vi "hatchPanelLoop.vi"() -> ()   [LabVIEW 2018]
uses:
  <vilib>/Platform/TimedLoop/XDataNode/timing_clust.ctl
  <vilib>/Platform/TimedLoop/XDataNode/nitl_modes.ctl
  <vilib>/Platform/TimedLoop/XDataNode/wakeup.ctl
  hatchPanelEnum.ctl
  HatchPanelMotionEnum.ctl
  HatchGrabPistonEnum.ctl
  hatchPanelNotifierCluster.ctl
  hatchPanelLockEnum.ctl
  hatchPanelStatemachineEnum.ctl
  stachModeHatchPanelStatemachineEnum.ctl
  hatchPanelClimbSMEnum.ctl
  <vilib>/platform/TimedLoop/XDataNode/XDataNode.xnode
  <vilib>/Platform/TimedLoop/XDataNode/XDNodeRunTimeDep.lvlib
  <userlib>/836-Library/System/TDMS_V2/Support/TDMS_DevRef.ctl
  <userlib>/836-Library/System/TDMS_V2/Support/Logging_Settings.ctl
  <userlib>/836-Library/System/TDMS_V2/Support/Group_FIFO_Config.ctl
  <userlib>/836-Library/System/TDMS_V2/Support/Channel_FIFO_Config.ctl
panel:
  in  "Tab Control":enum32{"Stach/OG", "Climb"}(tab)
  in  "hatchPanelSMGatherExtendTime":u32=380
  in  "hatchPanelSMScoreExtendTime":u32=700
  in  "hatchPanelSMGatherRetractTime":u32=650
  in  "hatchPanelSMScoreRetract":u32=500
  in  "hatchPanelSMReleaseTime":u32=150
  in  "hatchPanelSMGrabTime":u32=80
  in  "hatchPanelSMUnlockTime":u32=20
  in  "DistanceWantedFromTarget(Inch)":dbl=8.0
  in  "DistanceWantedAwayFromLoadingStation":dbl=-24.0
  out "Encoder Inches":dbl=-27.864021650326798
  in  "PanelDistanceDetect(V)":dbl=1.1
  in  "Wait for Unlock Time (ms)":u32=200
  in  "Wait for Extend Time (ms)":u32=1000
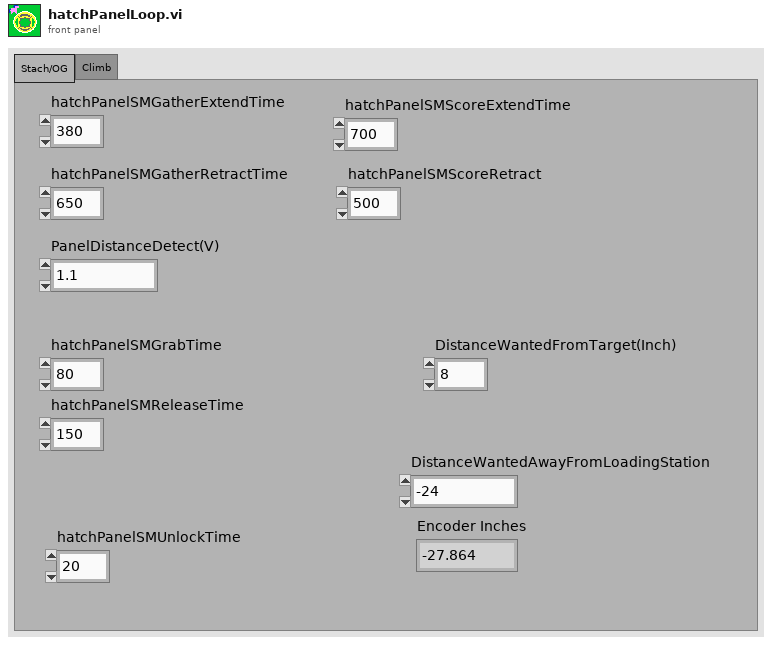
[diagram p1: front panel]
types:
  T1 = typedef "XDNodeRunTimeDep.lvlib/timing_clust.ctl" = cluster{"Expected End [f-1]":u64, "Actual End [f-1]":u64, "Finished Late? [f-1]":bool, "Expected End [i-1]":u64, "Actual End [i-1]":u64, "Finished Late? [i-1]":bool, "Expected Start [i]":u64, "Actual Start [i]":u64, "Expected Start [f]":u64, "Actual Start [f]":u64, "Source Name":string, "Structure Name":string, "Period":i64, "Deadline":i64, "Offset":i64, "Start":i64, "Priority":i32, "Timeout":i32, "Mode":T2, "Wakeup Reason":T3, "Error":errorcluster, "Source Type":string, "Secondary Source Type":string, "Global End Time":u64, "Global Start Time":u64, "Frame Duration":u64, "Iteration Duration":u64, "Assigned CPU":i32, "I/O Scan Engine Mode":u32}
  T2 = typedef "XDNodeRunTimeDep.lvlib/nitl_modes.ctl" = enum32{"No Change", "Process missed periods, maintain original phase", "Discard missed periods, maintain original phase", "Process missed periods, ignore original phase", "Discard missed periods, ignore original phase"}
  T3 = typedef "XDNodeRunTimeDep.lvlib/wakeup.ctl" = enum32{"Normal", "Aborted", "Asynchronous wakeup", "Timing source error", "Timed loop error", "Timeout"}
  T4 = typedef "WPI_SolenoidDevRef.ctl" = cluster{"DevStatus":errorcluster, "Pneumatics Control Module":u8, "Forward Solenoid Channel":T5, "Reverse Solenoid Channel":T5}
  T5 = typedef "WPI_SolenoidChannel.ctl" = enum8{"Solenoid 0", "Solenoid 1", "Solenoid 2", "Solenoid 3", "Solenoid 4", "Solenoid 5", "Solenoid 6", "Solenoid 7", "Invalid"}
  T6 = typedef "HatchGrabPistonEnum.ctl" = enum16{"Open", "Close"}
  T7 = typedef "HatchPanelMotionEnum.ctl" = enum16{"Retract", "Extend"}
  T8 = typedef "hatchPanelEnum.ctl" = enum16{"do nothing", "State Machine", "Stach Mode", "Climb Mode", "Retracted Closed", "Retracted Open", "Extended Closed", "Extended Open"}
  T9 = typedef "hatchPanelLockEnum.ctl" = enum16{"Unlocked", "Locked "}
  T10 = typedef "hatchPanelStatemachineEnum.ctl" = enum16{"Open to Gather", "Wait for Gather Extend", "Gather Extended", "Wait for Grab Panel", "Grab Panel", "Closed to Score", "Wait for Score Extend", "Ready to Score ", "Wait for Release Panel", "Release Panel", "Wait for Gather Retract", "Wait for Score Retract", "Wait for Gather Unlock", "Wait for Score Unlock", "Wait for Score Retract (Lock)", "Wait for Gather Retract (Lock)", "Gather End Lock", "Score End Lock"}
  T11 = typedef "stachModeHatchPanelStatemachineEnum.ctl" = enum16{"Stach Open to Gather", "Stach Wait for Gather Extend", "Stach Gather Extended", "Stach Wait for Grab Panel", "Stach Grab Panel", "Stach Closed to Score", "Stach Wait for Sonar Signal", "Stach Wait for Score Extend", "Stach Ready to Score ", "Stach Wait for Release Panel", "Stach Release Panel", "Stach Wait for Gather Retract", "Stach Wait for Score Retract", "Stach Wait for Gather Unlock", "Stach Wait for Score Unlock"}
  T12 = enum16{"Stach Open to Gather", "Stach Wait for Gather Extend", "Stach Gather Extended", "Stach Wait for Grab Panel", "Stach Grab Panel", "Stach Closed to Score", "Stach Wait for Sonar Signal", "Stach Wait for Score Extend", "Stach Ready to Score ", "Stach Wait for Release Panel", "Stach Release Panel", "Stach Wait for Gather Retract", "Stach Wait for Score Retract", "Stach Wait for Gather Unlock", "Stach Wait for Score Unlock", "Stach Gather End Lock", "Stach Score End Lock"}
  T13 = typedef "hatchPanelClimbSMEnum.ctl" = enum16{"Start", "Unlock", "Extend", "Ready for Climb", "Finished Climb"}
  T14 = typedef "hatchPanelNotifierCluster.ctl" = cluster{"Hatch Panel State":T8, "Mechanism Motion":bool, "Gathering Claw Motion":bool, "Scoring Claw Motion":bool}
  T15 = typedef "TDMS_DevRef.ctl" = cluster{"Name":string, "File Ref":refnum<k34>, "Start Time":timestamp, "Logging Settings":T16, "Group FIFO Config":T17[], "Data To Write":refnum<data-value>, "semaphore":T19, "Ref Time Reset":refnum<k4>}
  T16 = typedef "Logging_Settings.ctl" = cluster{"Data Grab Period":dbl, "File Write Period":dbl, "Max Stored Size":dbl, "Burst Size":dbl}
  T17 = typedef "Group_FIFO_Config.ctl" = cluster{"Group":string, "Channels":T18[], "Channel Names":string[]}
  T18 = typedef "Channel_FIFO_Config.ctl" = cluster{"Channel":string, "FIFO":refnum<k33>}
  T19 = typedef "Semaphore RefNum" = refnum<k1>
  T20 = typedef "WPI_MotorControlDeviceRef.ctl" = cluster{"DeviceStatus":errorcluster, "Type":T21, "PWM":cluster{"PWM Channel":T22, "DeadBand":T23}, "CAN":cluster{"Device Number":u8, "SetOutput VI Ref":variant, "GetOutput VI Ref":variant, "Enable VI Ref":variant, "Disable VI Ref":variant, "Data":variant}, "Invert":bool, "DIO PWM":cluster{"PWM \"Enable\" Channel":T22, "DIOChannel":T24, "PWM Rate":dbl}}
  T21 = typedef "WPI_MotorControlType.ctl" = enum16{"PWM", "CAN", "DIO PWM"}
  T22 = typedef "FPGA_DIOPWMChannel.ctl" = enum8{"PWM 0", "PWM 1", "PWM 2", "PWM 3", "PWM 4", "PWM 5", "PWM 6", "PWM 7", "PWM 8", "PWM 9", "PWM MXP 0", "PWM MXP 1", "PWM MXP 2", "PWM MXP 3", "PWM MXP 4", "PWM MXP 5", "PWM MXP 6", "PWM MXP 7", "PWM MXP 8", "PWM MXP 9", "Invalid"}
  T23 = typedef "WPI_PWMDeadband.ctl" = cluster{"Name":string, "maxPositivePwm":i32, "minPositivePwm":i32, "centerPwm":i32, "maxNegativePwm":i32, "minNegativePwm":i32, "angularRange":u16}
  T24 = typedef "FPGA_DIOChannel.ctl" = enum8{"DIO 0", "DIO 1", "DIO 2", "DIO 3", "DIO 4", "DIO 5", "DIO 6", "DIO 7", "DIO 8", "DIO 9", "DIO MXP 0", "DIO MXP 1", "DIO MXP 2", "DIO MXP 3", "DIO MXP 4", "DIO MXP 5", "DIO MXP 6", "DIO MXP 7", "DIO MXP 8", "DIO MXP 9", "DIO MXP 10", "DIO MXP 11", "DIO MXP 12", "DIO MXP 13", "DIO MXP 14", "DIO MXP 15", "SPI Port CS1", "SPI Port CS2", "SPI Port CS3", "SPI Port MISO", "SPI Port MOSI", "Invalid"}
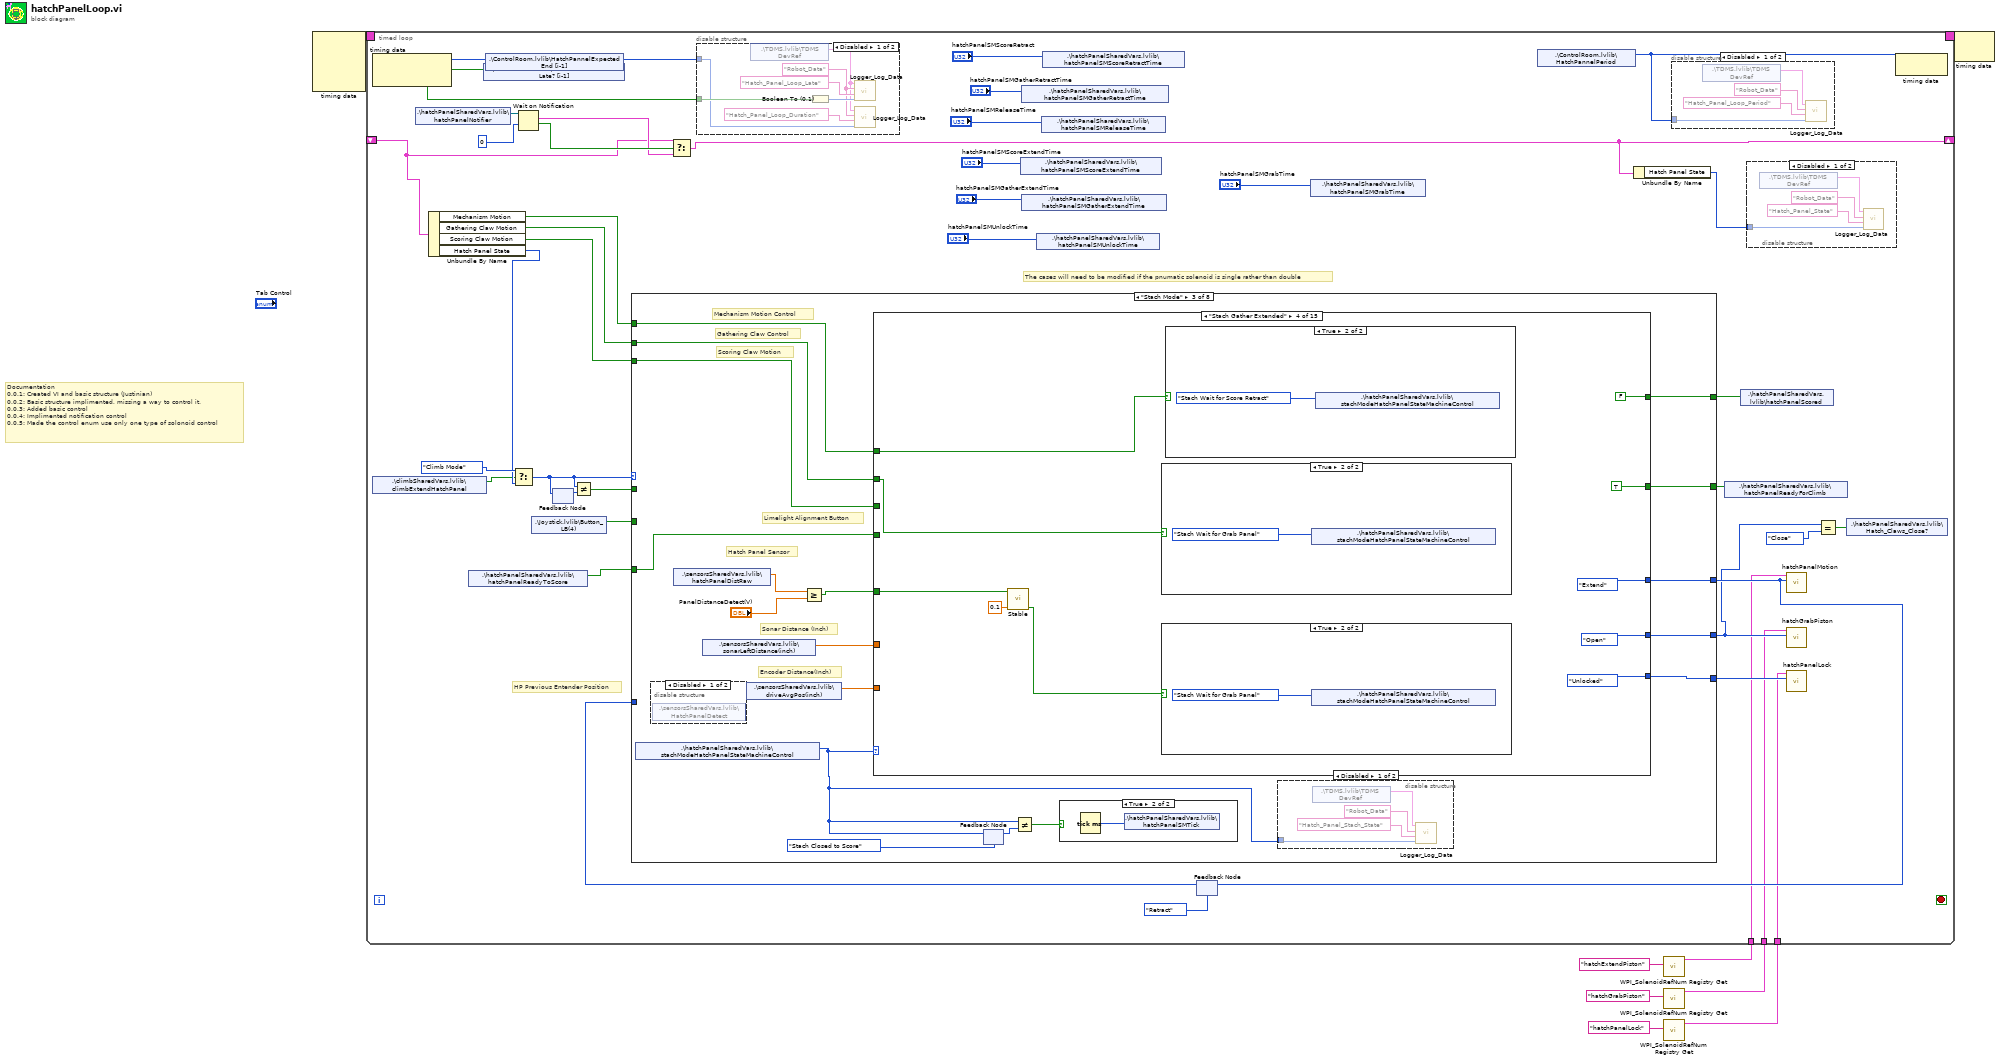
[diagram p0: block diagram]
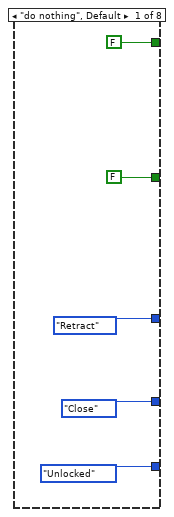
[diagram p5: hidden frame]
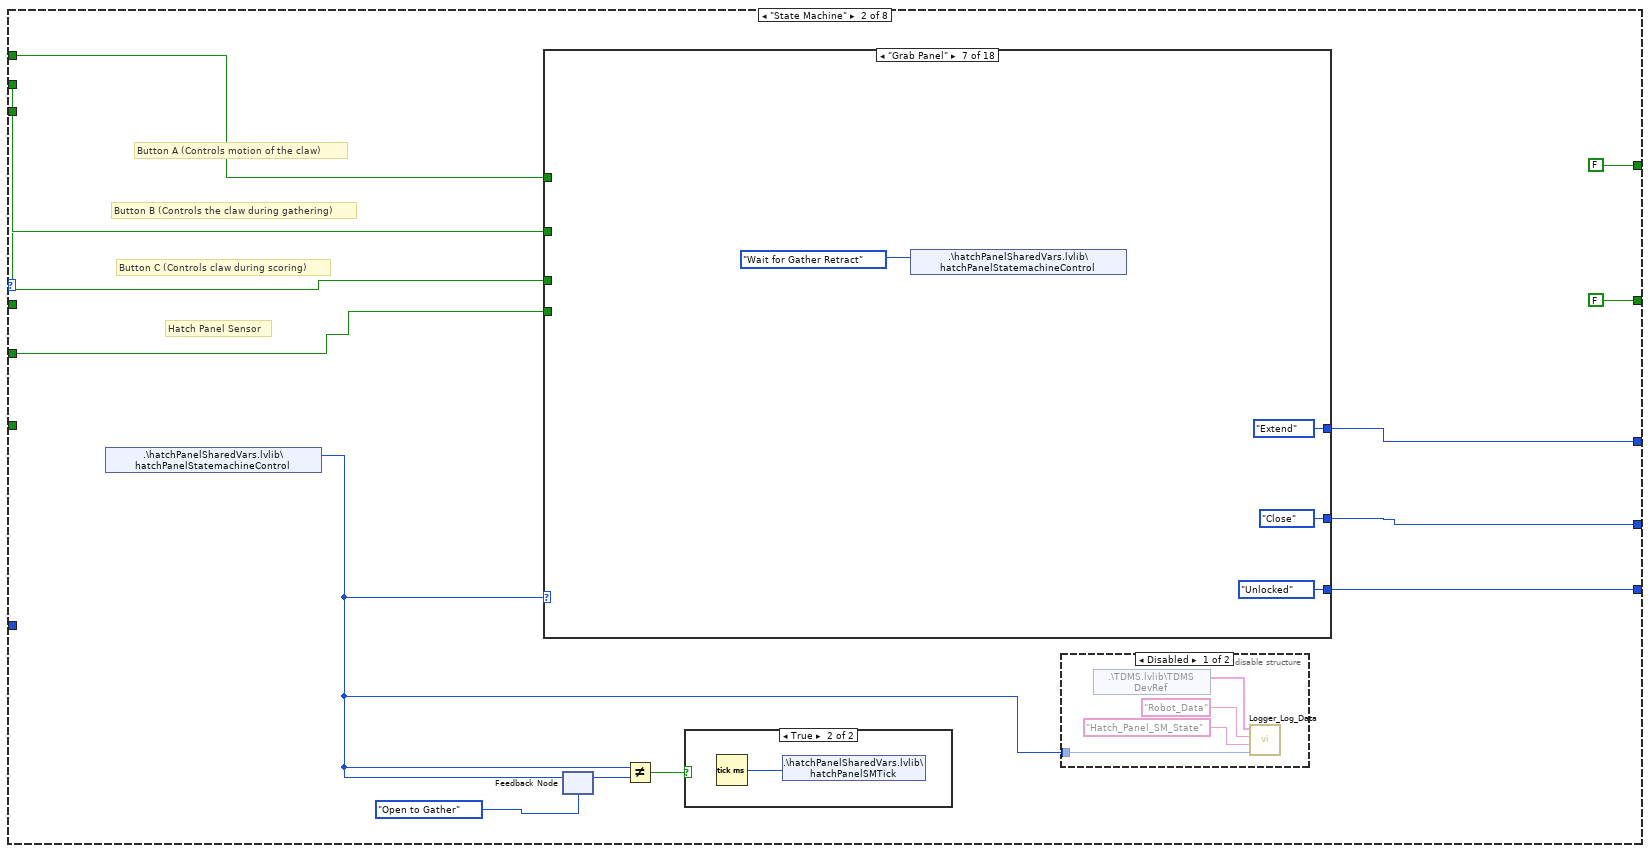
[diagram p6: hidden frame]
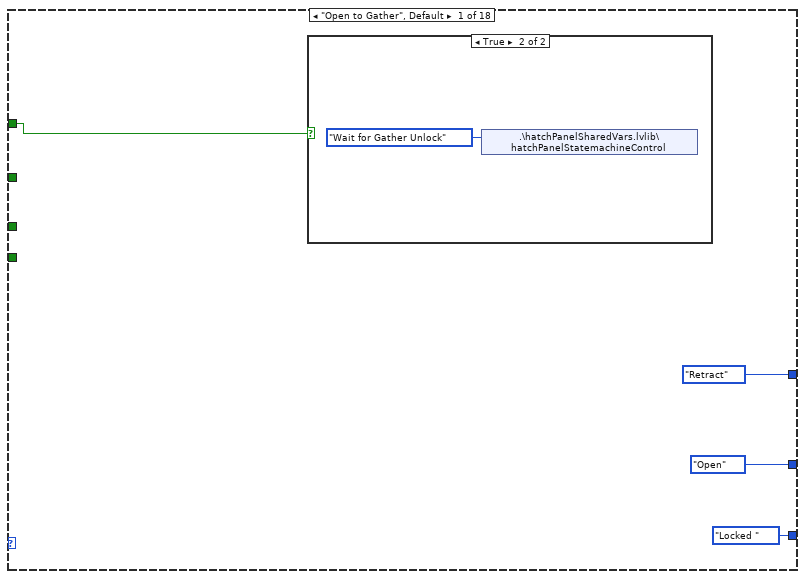
[diagram p9: hidden frame]
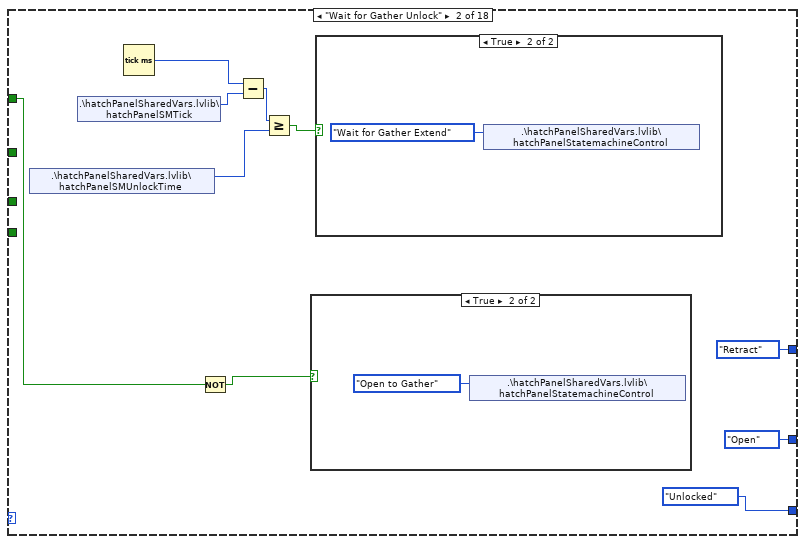
[diagram p11: hidden frame]
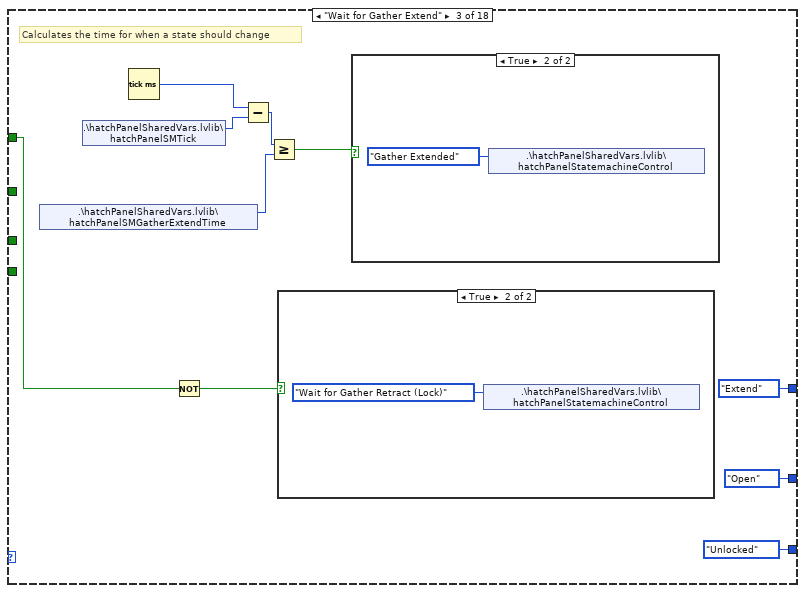
[diagram p14: hidden frame]
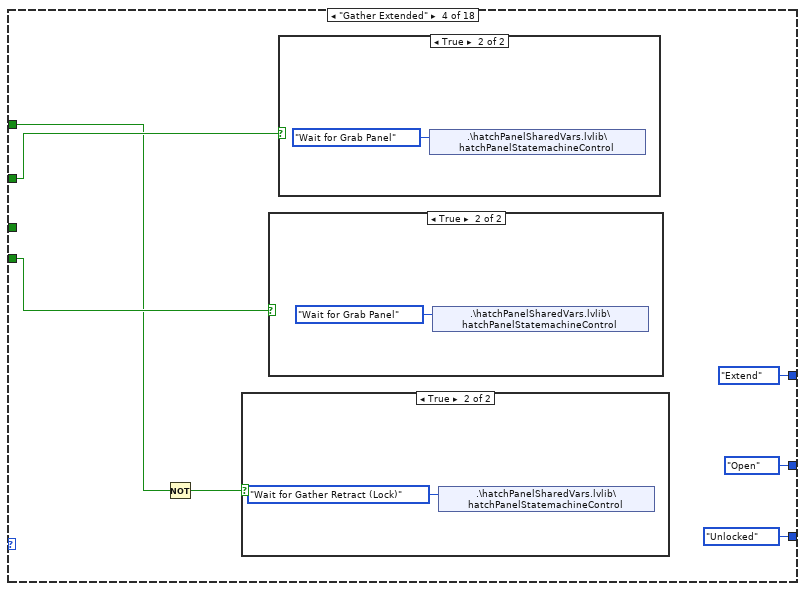
[diagram p17: hidden frame]
diagram:
  # "Documentation\n0.0.1: Created VI and basic structure (Justinian)\n0.0.2: Basic structure implimented, missing a way to control it.\n0.0.3: Added basic control\n0.0.4: Implimented notification control\n0.0.5: Made the control enum use only one type of solonoid control"
  n1 = node-c288() -> (w8:T1)  [unwired: 4 in]
  n2 = call <vilib>:"WPI_SolenoidRefNum Registry Get.vi"("refnum name"="hatchExtendPiston") -> ("SolenoidDevRef"=w3:T4)  [unwired: 9 in, 1 out]
  n3 = call <vilib>:"WPI_SolenoidRefNum Registry Get.vi"("refnum name"="hatchGrabPiston") -> ("SolenoidDevRef"=w2:T4)  [unwired: 9 in, 1 out]
  n4 = call <vilib>:"WPI_SolenoidRefNum Registry Get.vi"("refnum name"="hatchPanelLock") -> ("SolenoidDevRef"=w1:T4)  [unwired: 9 in, 1 out]
  n5 = timed-loop {
    timing: w8 -> [_]
    timing-out: [_] -> w7
    shift-right: [w17] -> _
    shift-left: _ -> [w18]
    tunnel: w3 -> [w12]
    tunnel: w2 -> [w11]
    tunnel: w1 -> [w10]
    stop <- _ stop-if-true
    # "HP Previous Entender Position"
    # "The cases will need to be modified if the pnumatic solenoid is single rather than double"
    n6 = node-c288() -> (w26:i64, w27:bool)  [unwired: 1 in]
    n7 = shared-variable ".\\climbSharedVars.lvlib\\climbExtendHatchPanel"() -> (w24:bool)  [unwired: 1 in, 1 out]
    n8 = shared-variable ".\\hatchPanelSharedVars.lvlib\\hatchPanelNotifier"() -> (w48:refnum<notifier>)  [unwired: 1 in, 1 out]
    n9 = Unbundle By Name(w18) -> ("Mechanism Motion"=w45:bool, "Gathering Claw Motion"=w44:bool, "Scoring Claw Motion"=w43:bool, "Hatch Panel State"=w31:T8)
    n10 = shared-variable ".\\hatchPanelSharedVars.lvlib\\hatchPanelReadyToScore"() -> (w20:bool)  [unwired: 1 in, 1 out]
    n11 = shared-variable ".\\ControlRoom.lvlib\\HatchPannelFinished Late? [i-1]"(w27) -> ()  [unwired: 1 in, 1 out]
    n12 = shared-variable ".\\ControlRoom.lvlib\\HatchPannelExpected End [i-1]"(w26) -> ()  [unwired: 1 in, 1 out]
    n13 = Select(t=hatchPanelEnum."Climb Mode", s=w24, f=w31) -> (s? t:f=w30:T8)
    n14 = Wait on Notification(notifier=w48, timeout in ms (-1)=0) -> (notification=w19:T14, timed out?=w47:bool)  [unwired: 2 in, 2 out]
    n15 = shared-variable ".\\Joystick.lvlib\\Button_LB(4)"() -> (w42:bool)  [unwired: 1 in, 1 out]
    n16 = feedback #1() -> (w33:T8)  [unwired: 1 in]
    n17 = feedback-in #1(w30) -> ()
    n18 = Not Equal?(x=w30, y=w33) -> (x != y?=w29:bool)
    n19 = Select(t=w18, s=w47, f=w19) -> (s? t:f=w17:T14)
    n20 = disable-structure shown="Disabled" {
      disable-tunnel: w27 -> [w63 _]
      disable-tunnel: w26 -> [w62 _]
      frame Disabled {
        w58 = "Robot_Data" ("Group")
        n21 = shared-variable ".\\TDMS.lvlib\\TDMS DevRef"() -> (w57:T15)  [unwired: 1 in, 1 out]
        n22 = Boolean To (0,1)(Boolean=w63) -> (0, 1=w60:i16)
        n23 = call <userlib>:"Logger_Log_Data.vi"("Data"=w60, "Channel"="Hatch_Panel_Loop_Late", "Group"=w58, "TDMS DevRef"=w57) -> ()  [unwired: 7 in, 1 out]
        n24 = call <userlib>:"Logger_Log_Data.vi"("Data"=w62, "Channel"="Hatch_Panel_Loop_Duration", "Group"=w58, "TDMS DevRef"=w57) -> ()  [unwired: 7 in, 1 out]
      }
      frame Enabled {
      }
    }
    n25 = shared-variable ".\\hatchPanelSharedVars.lvlib\\hatchPanelSMScoreExtendTime"("hatchPanelSMScoreExtendTime") -> ()  [unwired: 1 in, 1 out]
    n26 = shared-variable ".\\hatchPanelSharedVars.lvlib\\hatchPanelSMGatherRetractTime"("hatchPanelSMGatherRetractTime") -> ()  [unwired: 1 in, 1 out]
    n27 = shared-variable ".\\hatchPanelSharedVars.lvlib\\hatchPanelSMGatherExtendTime"("hatchPanelSMGatherExtendTime") -> ()  [unwired: 1 in, 1 out]
    n28 = shared-variable ".\\hatchPanelSharedVars.lvlib\\hatchPanelSMUnlockTime"("hatchPanelSMUnlockTime") -> ()  [unwired: 1 in, 1 out]
    n29 = shared-variable ".\\hatchPanelSharedVars.lvlib\\hatchPanelSMReleaseTime"("hatchPanelSMReleaseTime") -> ()  [unwired: 1 in, 1 out]
    n30 = shared-variable ".\\hatchPanelSharedVars.lvlib\\hatchPanelSMScoreRetractTime"("hatchPanelSMScoreRetract") -> ()  [unwired: 1 in, 1 out]
    n31 = feedback #2(HatchPanelMotionEnum."Retract") -> (w21:T7)
    n32 = case shown="\"Stach Mode\"" w30 {
      tunnel: w45 -> [_ w80 w245 _ _ _ _ _]
      tunnel: w44 -> [_ w79 w244 _ _ _ _ _]
      tunnel: w43 -> [_ w78 w243 _ _ _ _ _]
      tunnel: [HatchPanelMotionEnum."Retract" w75 w251 w454 HatchPanelMotionEnum."Retract" HatchPanelMotionEnum."Retract" HatchPanelMotionEnum."Extend" HatchPanelMotionEnum."Extend"] -> w23
      tunnel: [HatchGrabPistonEnum."Close" w74 w250 w453 HatchGrabPistonEnum."Close" HatchGrabPistonEnum."Open" HatchGrabPistonEnum."Close" HatchGrabPistonEnum."Open"] -> w13
      tunnel: w42 -> [_ w73 _ _ _ _ _ _]
      tunnel: [hatchPanelLockEnum."Unlocked" w72 w249 w452 hatchPanelLockEnum."Unlocked" hatchPanelLockEnum."Unlocked" hatchPanelLockEnum."Unlocked" hatchPanelLockEnum."Unlocked"] -> w36
      tunnel: w29 -> [_ _ _ w455 _ _ _ _]
      tunnel: [FALSE FALSE w239 w451 FALSE FALSE FALSE FALSE] -> w28
      tunnel: w21 -> [_ _ _ w446 _ _ _ _]
      tunnel: w20 -> [_ _ w238 _ _ _ _ _]
      tunnel: [FALSE FALSE w237 FALSE FALSE FALSE FALSE FALSE] -> w9
      frame "do nothing", Default {
      }
      frame "State Machine" {
        # "Hatch Panel Sensor"
        # "Button C (Controls claw during scoring)"
        # "Button B (Controls the claw during gathering)"
        # "Button A (Controls motion of the claw)"
        n33 = shared-variable ".\\hatchPanelSharedVars.lvlib\\hatchPanelStatemachineControl"() -> (w70:T10)  [unwired: 1 in, 1 out]
        n34 = case shown="\"Grab Panel\"" w70 {
          tunnel: [HatchGrabPistonEnum."Open" HatchGrabPistonEnum."Open" HatchGrabPistonEnum."Open" HatchGrabPistonEnum."Open" HatchGrabPistonEnum."Open" HatchGrabPistonEnum."Close" HatchGrabPistonEnum."Close" HatchGrabPistonEnum."Close" HatchGrabPistonEnum."Close" HatchGrabPistonEnum."Close" HatchGrabPistonEnum."Close" HatchGrabPistonEnum."Close" HatchGrabPistonEnum."Close" HatchGrabPistonEnum."Open" HatchGrabPistonEnum."Open" HatchGrabPistonEnum."Open" HatchGrabPistonEnum."Close" HatchGrabPistonEnum."Open"] -> w74
          tunnel: [HatchPanelMotionEnum."Retract" HatchPanelMotionEnum."Retract" HatchPanelMotionEnum."Extend" HatchPanelMotionEnum."Extend" HatchPanelMotionEnum."Retract" HatchPanelMotionEnum."Extend" HatchPanelMotionEnum."Extend" HatchPanelMotionEnum."Retract" HatchPanelMotionEnum."Retract" HatchPanelMotionEnum."Retract" HatchPanelMotionEnum."Extend" HatchPanelMotionEnum."Retract" HatchPanelMotionEnum."Extend" HatchPanelMotionEnum."Extend" HatchPanelMotionEnum."Extend" HatchPanelMotionEnum."Retract" HatchPanelMotionEnum."Retract" HatchPanelMotionEnum."Retract"] -> w75
          tunnel: w73 -> [_ _ _ w120 _ _ _ _ _ _ _ _ _ _ _ _ _ _]
          tunnel: w78 -> [_ _ _ _ _ _ _ _ _ _ _ _ w195 _ _ _ _ _]
          tunnel: w80 -> [w88 w92 w106 w118 _ _ _ _ w158 _ w173 _ w194 _ _ _ w223 w232]
          tunnel: w79 -> [_ _ _ w119 _ _ _ _ _ _ _ _ _ _ _ _ _ _]
          tunnel: [hatchPanelLockEnum."Locked " hatchPanelLockEnum."Unlocked" hatchPanelLockEnum."Unlocked" hatchPanelLockEnum."Unlocked" hatchPanelLockEnum."Unlocked" hatchPanelLockEnum."Unlocked" hatchPanelLockEnum."Unlocked" hatchPanelLockEnum."Unlocked" hatchPanelLockEnum."Locked " hatchPanelLockEnum."Unlocked" hatchPanelLockEnum."Unlocked" hatchPanelLockEnum."Unlocked" hatchPanelLockEnum."Unlocked" hatchPanelLockEnum."Unlocked" hatchPanelLockEnum."Unlocked" hatchPanelLockEnum."Unlocked" hatchPanelLockEnum."Unlocked" hatchPanelLockEnum."Unlocked"] -> w72
          frame "Open to Gather", Default {
            n35 = case shown="True" w88 {
              frame False {
              }
              frame True {
                n36 = shared-variable ".\\hatchPanelSharedVars.lvlib\\hatchPanelStatemachineControl"(hatchPanelStatemachineEnum."Wait for Gather Unlock" ("hatchPanelStatemachineControl")) -> ()  [unwired: 1 in, 1 out]
              }
            }
          }
          frame "Wait for Gather Unlock" {
            n37 = shared-variable ".\\hatchPanelSharedVars.lvlib\\hatchPanelSMUnlockTime"() -> (w97:u32)  [unwired: 1 in, 1 out]
            n38 = shared-variable ".\\hatchPanelSharedVars.lvlib\\hatchPanelSMTick"() -> (w101:u32)  [unwired: 1 in, 1 out]
            n39 = Tick Count (ms)() -> (millisecond timer value=w100:u32)
            n40 = Not(x=w92) -> (.not. x?=w93:bool)
            n41 = Subtract(x=w100, y=w101) -> (x-y=w99:u32)
            n42 = Greater Or Equal?(x=w99, y=w97) -> (x >= y?=w98:bool)
            n43 = case shown="True" w93 {
              frame False {
              }
              frame True {
                n44 = shared-variable ".\\hatchPanelSharedVars.lvlib\\hatchPanelStatemachineControl"(hatchPanelStatemachineEnum."Open to Gather" ("hatchPanelStatemachineControl")) -> ()  [unwired: 1 in, 1 out]
              }
            }
            n45 = case shown="True" w98 {
              frame False {
              }
              frame True {
                n46 = shared-variable ".\\hatchPanelSharedVars.lvlib\\hatchPanelStatemachineControl"(hatchPanelStatemachineEnum."Wait for Gather Extend" ("hatchPanelStatemachineControl")) -> ()  [unwired: 1 in, 1 out]
              }
            }
          }
          frame "Wait for Gather Extend" {
            # "Calculates the time for when a state should change"
            n47 = shared-variable ".\\hatchPanelSharedVars.lvlib\\hatchPanelSMGatherExtendTime"() -> (w108:u32)  [unwired: 1 in, 1 out]
            n48 = shared-variable ".\\hatchPanelSharedVars.lvlib\\hatchPanelSMTick"() -> (w111:u32)  [unwired: 1 in, 1 out]
            n49 = Tick Count (ms)() -> (millisecond timer value=w110:u32)
            n50 = Not(x=w106) -> (.not. x?=w105:bool)
            n51 = Subtract(x=w110, y=w111) -> (x-y=w109:u32)
            n52 = Greater Or Equal?(x=w109, y=w108) -> (x >= y?=w107:bool)
            n53 = case shown="True" w105 {
              frame False {
              }
              frame True {
                n54 = shared-variable ".\\hatchPanelSharedVars.lvlib\\hatchPanelStatemachineControl"(hatchPanelStatemachineEnum."Wait for Gather Retract (Lock)" ("hatchPanelStatemachineControl")) -> ()  [unwired: 1 in, 1 out]
              }
            }
            n55 = case shown="True" w107 {
              frame False {
              }
              frame True {
                n56 = shared-variable ".\\hatchPanelSharedVars.lvlib\\hatchPanelStatemachineControl"(hatchPanelStatemachineEnum."Gather Extended" ("hatchPanelStatemachineControl")) -> ()  [unwired: 1 in, 1 out]
              }
            }
          }
          frame "Gather Extended" {
            n57 = Not(x=w118) -> (.not. x?=w117:bool)
            n58 = case shown="True" w117 {
              frame False {
              }
              frame True {
                n59 = shared-variable ".\\hatchPanelSharedVars.lvlib\\hatchPanelStatemachineControl"(hatchPanelStatemachineEnum."Wait for Gather Retract (Lock)" ("hatchPanelStatemachineControl")) -> ()  [unwired: 1 in, 1 out]
              }
            }
            n60 = case shown="True" w120 {
              frame False {
              }
              frame True {
                n61 = shared-variable ".\\hatchPanelSharedVars.lvlib\\hatchPanelStatemachineControl"(hatchPanelStatemachineEnum."Wait for Grab Panel" ("hatchPanelStatemachineControl")) -> ()  [unwired: 1 in, 1 out]
              }
            }
            n62 = case shown="True" w119 {
              frame False {
              }
              frame True {
                n63 = shared-variable ".\\hatchPanelSharedVars.lvlib\\hatchPanelStatemachineControl"(hatchPanelStatemachineEnum."Wait for Grab Panel" ("hatchPanelStatemachineControl")) -> ()  [unwired: 1 in, 1 out]
              }
            }
          }
          frame "Wait for Gather Retract (Lock)" {
            n64 = shared-variable ".\\hatchPanelSharedVars.lvlib\\hatchPanelSMGatherRetractTime"() -> (w129:u32)  [unwired: 1 in, 1 out]
            n65 = shared-variable ".\\hatchPanelSharedVars.lvlib\\hatchPanelSMTick"() -> (w133:u32)  [unwired: 1 in, 1 out]
            n66 = Tick Count (ms)() -> (millisecond timer value=w132:u32)
            n67 = Subtract(x=w132, y=w133) -> (x-y=w131:u32)
            n68 = Greater Or Equal?(x=w131, y=w129) -> (x >= y?=w130:bool)
            n69 = case shown="True" w130 {
              frame False {
              }
              frame True {
                n70 = shared-variable ".\\hatchPanelSharedVars.lvlib\\hatchPanelStatemachineControl"(hatchPanelStatemachineEnum."Open to Gather" ("hatchPanelStatemachineControl")) -> ()  [unwired: 1 in, 1 out]
              }
            }
          }
          frame "Wait for Grab Panel" {
            n71 = shared-variable ".\\hatchPanelSharedVars.lvlib\\hatchPanelSMGrabTime"() -> (w135:u32)  [unwired: 1 in, 1 out]
            n72 = shared-variable ".\\hatchPanelSharedVars.lvlib\\hatchPanelSMTick"() -> (w140:u32)  [unwired: 1 in, 1 out]
            n73 = Tick Count (ms)() -> (millisecond timer value=w139:u32)
            n74 = Subtract(x=w139, y=w140) -> (x-y=w137:u32)
            n75 = Greater Or Equal?(x=w137, y=w135) -> (x >= y?=w138:bool)
            n76 = case shown="True" w138 {
              frame False {
              }
              frame True {
                n77 = shared-variable ".\\hatchPanelSharedVars.lvlib\\hatchPanelStatemachineControl"(hatchPanelStatemachineEnum."Grab Panel" ("hatchPanelStatemachineControl")) -> ()  [unwired: 1 in, 1 out]
              }
            }
          }
          frame "Grab Panel" {
            n78 = shared-variable ".\\hatchPanelSharedVars.lvlib\\hatchPanelStatemachineControl"(hatchPanelStatemachineEnum."Wait for Gather Retract" ("hatchPanelStatemachineControl")) -> ()  [unwired: 1 in, 1 out]
          }
          frame "Wait for Gather Retract" {
            n79 = shared-variable ".\\hatchPanelSharedVars.lvlib\\hatchPanelSMGatherRetractTime"() -> (w150:u32)  [unwired: 1 in, 1 out]
            n80 = shared-variable ".\\hatchPanelSharedVars.lvlib\\hatchPanelSMTick"() -> (w153:u32)  [unwired: 1 in, 1 out]
            n81 = Tick Count (ms)() -> (millisecond timer value=w152:u32)
            n82 = Subtract(x=w152, y=w153) -> (x-y=w151:u32)
            n83 = Greater Or Equal?(x=w151, y=w150) -> (x >= y?=w148:bool)
            n84 = case shown="True" w148 {
              frame False {
              }
              frame True {
                n85 = shared-variable ".\\hatchPanelSharedVars.lvlib\\hatchPanelStatemachineControl"(hatchPanelStatemachineEnum."Gather End Lock" ("hatchPanelStatemachineControl")) -> ()  [unwired: 1 in, 1 out]
              }
            }
          }
          frame "Closed to Score" {
            n86 = case shown="True" w158 {
              frame False {
              }
              frame True {
                n87 = shared-variable ".\\hatchPanelSharedVars.lvlib\\hatchPanelStatemachineControl"(hatchPanelStatemachineEnum."Wait for Score Unlock" ("hatchPanelStatemachineControl")) -> ()  [unwired: 1 in, 1 out]
              }
            }
          }
          frame "Wait for Score Unlock" {
            n88 = shared-variable ".\\hatchPanelSharedVars.lvlib\\hatchPanelSMUnlockTime"() -> (w162:u32)  [unwired: 1 in, 1 out]
            n89 = shared-variable ".\\hatchPanelSharedVars.lvlib\\hatchPanelSMTick"() -> (w169:u32)  [unwired: 1 in, 1 out]
            n90 = Tick Count (ms)() -> (millisecond timer value=w168:u32)
            n91 = Subtract(x=w168, y=w169) -> (x-y=w167:u32)
            n92 = Greater Or Equal?(x=w167, y=w162) -> (x >= y?=w166:bool)
            n93 = case shown="True" w166 {
              frame False {
              }
              frame True {
                n94 = shared-variable ".\\hatchPanelSharedVars.lvlib\\hatchPanelStatemachineControl"(hatchPanelStatemachineEnum."Wait for Score Extend" ("hatchPanelStatemachineControl")) -> ()  [unwired: 1 in, 1 out]
              }
            }
          }
          frame "Wait for Score Extend" {
            n95 = shared-variable ".\\hatchPanelSharedVars.lvlib\\hatchPanelSMTick"() -> (w178:u32)  [unwired: 1 in, 1 out]
            n96 = shared-variable ".\\hatchPanelSharedVars.lvlib\\hatchPanelSMScoreExtendTime"() -> (w174:u32)  [unwired: 1 in, 1 out]
            n97 = Tick Count (ms)() -> (millisecond timer value=w177:u32)
            n98 = Not(x=w173) -> (.not. x?=w172:bool)
            n99 = Subtract(x=w177, y=w178) -> (x-y=w176:u32)
            n100 = case shown="True" w172 {
              frame False {
              }
              frame True {
                n101 = shared-variable ".\\hatchPanelSharedVars.lvlib\\hatchPanelStatemachineControl"(hatchPanelStatemachineEnum."Wait for Score Retract (Lock)" ("hatchPanelStatemachineControl")) -> ()  [unwired: 1 in, 1 out]
              }
            }
            n102 = Greater Or Equal?(x=w176, y=w174) -> (x >= y?=w175:bool)
            n103 = case shown="True" w175 {
              frame False {
              }
              frame True {
                n104 = shared-variable ".\\hatchPanelSharedVars.lvlib\\hatchPanelStatemachineControl"(hatchPanelStatemachineEnum."Ready to Score " ("hatchPanelStatemachineControl")) -> ()  [unwired: 1 in, 1 out]
              }
            }
          }
          frame "Wait for Score Retract (Lock)" {
            n105 = shared-variable ".\\hatchPanelSharedVars.lvlib\\hatchPanelSMScoreRetractTime"() -> (w183:u32)  [unwired: 1 in, 1 out]
            n106 = shared-variable ".\\hatchPanelSharedVars.lvlib\\hatchPanelSMTick"() -> (w190:u32)  [unwired: 1 in, 1 out]
            n107 = Tick Count (ms)() -> (millisecond timer value=w189:u32)
            n108 = Subtract(x=w189, y=w190) -> (x-y=w188:u32)
            n109 = Greater Or Equal?(x=w188, y=w183) -> (x >= y?=w187:bool)
            n110 = case shown="True" w187 {
              frame False {
              }
              frame True {
                n111 = shared-variable ".\\hatchPanelSharedVars.lvlib\\hatchPanelStatemachineControl"(hatchPanelStatemachineEnum."Closed to Score" ("hatchPanelStatemachineControl")) -> ()  [unwired: 1 in, 1 out]
              }
            }
          }
          frame "Ready to Score " {
            n112 = Not(x=w194) -> (.not. x?=w193:bool)
            n113 = case shown="True" w193 {
              frame False {
              }
              frame True {
                n114 = shared-variable ".\\hatchPanelSharedVars.lvlib\\hatchPanelStatemachineControl"(hatchPanelStatemachineEnum."Wait for Score Retract (Lock)" ("hatchPanelStatemachineControl")) -> ()  [unwired: 1 in, 1 out]
              }
            }
            n115 = case shown="True" w195 {
              frame False {
              }
              frame True {
                n116 = shared-variable ".\\hatchPanelSharedVars.lvlib\\hatchPanelStatemachineControl"(hatchPanelStatemachineEnum."Wait for Release Panel" ("hatchPanelStatemachineControl")) -> ()  [unwired: 1 in, 1 out]
              }
            }
          }
          frame "Wait for Release Panel" {
            n117 = shared-variable ".\\hatchPanelSharedVars.lvlib\\hatchPanelSMReleaseTime"() -> (w201:u32)  [unwired: 1 in, 1 out]
            n118 = shared-variable ".\\hatchPanelSharedVars.lvlib\\hatchPanelSMTick"() -> (w205:u32)  [unwired: 1 in, 1 out]
            n119 = Tick Count (ms)() -> (millisecond timer value=w204:u32)
            n120 = Subtract(x=w204, y=w205) -> (x-y=w203:u32)
            n121 = Greater Or Equal?(x=w203, y=w201) -> (x >= y?=w202:bool)
            n122 = case shown="True" w202 {
              frame False {
              }
              frame True {
                n123 = shared-variable ".\\hatchPanelSharedVars.lvlib\\hatchPanelStatemachineControl"(hatchPanelStatemachineEnum."Release Panel" ("hatchPanelStatemachineControl")) -> ()  [unwired: 1 in, 1 out]
              }
            }
          }
          frame "Release Panel" {
            n124 = shared-variable ".\\hatchPanelSharedVars.lvlib\\hatchPanelStatemachineControl"(hatchPanelStatemachineEnum."Wait for Score Retract" ("hatchPanelStatemachineControl")) -> ()  [unwired: 1 in, 1 out]
          }
          frame "Wait for Score Retract" {
            n125 = shared-variable ".\\hatchPanelSharedVars.lvlib\\hatchPanelSMScoreRetractTime"() -> (w215:u32)  [unwired: 1 in, 1 out]
            n126 = shared-variable ".\\hatchPanelSharedVars.lvlib\\hatchPanelSMTick"() -> (w218:u32)  [unwired: 1 in, 1 out]
            n127 = Tick Count (ms)() -> (millisecond timer value=w217:u32)
            n128 = Subtract(x=w217, y=w218) -> (x-y=w216:u32)
            n129 = Greater Or Equal?(x=w216, y=w215) -> (x >= y?=w213:bool)
            n130 = case shown="True" w213 {
              frame False {
              }
              frame True {
                n131 = shared-variable ".\\hatchPanelSharedVars.lvlib\\hatchPanelStatemachineControl"(hatchPanelStatemachineEnum."Score End Lock" ("hatchPanelStatemachineControl")) -> ()  [unwired: 1 in, 1 out]
              }
            }
          }
          frame "Gather End Lock" {
            n132 = Not(x=w223) -> (.not. x?=w222:bool)
            n133 = case shown="True" w222 {
              frame False {
              }
              frame True {
                n134 = shared-variable ".\\hatchPanelSharedVars.lvlib\\hatchPanelStatemachineControl"(hatchPanelStatemachineEnum."Closed to Score" ("hatchPanelStatemachineControl")) -> ()  [unwired: 1 in, 1 out]
              }
            }
          }
          frame "Score End Lock" {
            n135 = Not(x=w232) -> (.not. x?=w231:bool)
            n136 = case shown="True" w231 {
              frame False {
              }
              frame True {
                n137 = shared-variable ".\\hatchPanelSharedVars.lvlib\\hatchPanelStatemachineControl"(hatchPanelStatemachineEnum."Open to Gather" ("hatchPanelStatemachineControl")) -> ()  [unwired: 1 in, 1 out]
              }
            }
          }
        }
        n138 = feedback-in #3(w70) -> ()
        n139 = feedback #3(hatchPanelStatemachineEnum."Open to Gather" ("Enum")) -> (w77:T10)
        n140 = Not Equal?(x=w70, y=w77) -> (x != y?=w81:bool)
        n141 = case shown="True" w81 {
          frame False {
          }
          frame True {
            n142 = Tick Count (ms)() -> (millisecond timer value=w86:u32)
            n143 = shared-variable ".\\hatchPanelSharedVars.lvlib\\hatchPanelSMTick"(w86) -> ()  [unwired: 1 in, 1 out]
          }
        }
        n144 = disable-structure shown="Disabled" {
          disable-tunnel: w70 -> [w85 _]
          frame Disabled {
            n145 = shared-variable ".\\TDMS.lvlib\\TDMS DevRef"() -> (w83:T15)  [unwired: 1 in, 1 out]
            n146 = call <userlib>:"Logger_Log_Data.vi"("Data"=w85, "Channel"="Hatch_Panel_SM_State", "Group"="Robot_Data", "TDMS DevRef"=w83) -> ()  [unwired: 7 in, 1 out]
          }
          frame Enabled {
          }
        }
      }
      frame "Stach Mode" {
        # "Encoder Distance(Inch)"
        # "Sonar Distance (Inch)"
        # "Hatch Panel Sensor"
        # "Scoring Claw Motion"
        # "Gathering Claw Control"
        # "Mechanism Motion Control"
        # "Limelight Alignment Button"
        n147 = shared-variable ".\\hatchPanelSharedVars.lvlib\\stachModeHatchPanelStateMachineControl"() -> (w240:T12)  [unwired: 1 in, 1 out]
        n148 = disable-structure shown="Disabled" {
          frame Disabled {
            n149 = shared-variable ".\\sensorsSharedVars.lvlib\\HatchPanelDetect"() -> ()  [unwired: 1 in, 2 out]
          }
          frame Enabled {
          }
        }
        n150 = shared-variable ".\\sensorsSharedVars.lvlib\\hatchPanelDistRaw"() -> (w235:dbl)  [unwired: 1 in, 1 out]
        n151 = shared-variable ".\\sensorsSharedVars.lvlib\\sonarLeftDistance(inch)"() -> (w242:dbl)  [unwired: 1 in, 1 out]
        n152 = shared-variable ".\\sensorsSharedVars.lvlib\\driveAvgPos(inch)"() -> (w241:dbl)  [unwired: 1 in, 1 out]
        n153 = Greater Or Equal?(x=w235, y="PanelDistanceDetect(V)") -> (x >= y?=w234:bool)
        n154 = case shown="\"Stach Gather Extended\"" w240 {
          tunnel: [HatchPanelMotionEnum."Retract" HatchPanelMotionEnum."Retract" HatchPanelMotionEnum."Extend" HatchPanelMotionEnum."Extend" HatchPanelMotionEnum."Extend" HatchPanelMotionEnum."Extend" HatchPanelMotionEnum."Retract" HatchPanelMotionEnum."Retract" HatchPanelMotionEnum."Retract" HatchPanelMotionEnum."Retract" HatchPanelMotionEnum."Extend" HatchPanelMotionEnum."Extend" HatchPanelMotionEnum."Extend" HatchPanelMotionEnum."Extend" HatchPanelMotionEnum."Retract"] -> w251
          tunnel: [HatchGrabPistonEnum."Open" HatchGrabPistonEnum."Open" HatchGrabPistonEnum."Open" HatchGrabPistonEnum."Open" HatchGrabPistonEnum."Close" HatchGrabPistonEnum."Close" HatchGrabPistonEnum."Close" HatchGrabPistonEnum."Close" HatchGrabPistonEnum."Close" HatchGrabPistonEnum."Close" HatchGrabPistonEnum."Close" HatchGrabPistonEnum."Close" HatchGrabPistonEnum."Open" HatchGrabPistonEnum."Open" HatchGrabPistonEnum."Open"] -> w250
          tunnel: [hatchPanelLockEnum."Locked " hatchPanelLockEnum."Unlocked" hatchPanelLockEnum."Unlocked" hatchPanelLockEnum."Unlocked" hatchPanelLockEnum."Unlocked" hatchPanelLockEnum."Unlocked" hatchPanelLockEnum."Unlocked" hatchPanelLockEnum."Locked " hatchPanelLockEnum."Locked " hatchPanelLockEnum."Unlocked" hatchPanelLockEnum."Unlocked" hatchPanelLockEnum."Unlocked" hatchPanelLockEnum."Unlocked" hatchPanelLockEnum."Unlocked" hatchPanelLockEnum."Unlocked"] -> w249
          tunnel: w238 -> [w263 _ _ _ _ _ _ w356 w370 _ _ _ _ _ _]
          tunnel: w245 -> [w262 _ _ w297 _ w330 _ w355 w373 _ _ w409 _ _ _]
          tunnel: w244 -> [_ _ _ w298 _ w329 _ _ _ _ _ _ _ _ _]
          tunnel: w243 -> [_ _ _ _ _ _ _ _ _ _ _ w406 _ _ _]
          tunnel: w234 -> [w258 _ _ w294 _ _ _ w353 _ _ _ _ _ _ _]
          tunnel: w242 -> [_ _ _ _ _ _ _ _ w365 _ _ _ _ _ _]
          tunnel: w241 -> [_ _ _ _ w305 w323 _ _ _ _ _ _ _ _ _]
          tunnel: [FALSE FALSE FALSE TRUE FALSE FALSE FALSE FALSE FALSE FALSE FALSE FALSE FALSE FALSE FALSE] -> w239
          tunnel: [FALSE FALSE FALSE FALSE FALSE FALSE FALSE FALSE FALSE FALSE FALSE FALSE TRUE TRUE FALSE] -> w237
          frame "Stach Open to Gather", Default {
            n155 = call <userlib>:"Stable.vi"("Eval Period (sec)"=1.0, "Signal Input"=w258) -> ("Stable"=w259:bool)  [unwired: 9 in]
            n156 = case shown="True" w262 {
              frame False {
              }
              frame True {
                (unwired) stachModeHatchPanelStatemachineEnum."Stach Wait for Gather Unlock" ("Hatch Panel State")
                n157 = shared-variable ".\\hatchPanelSharedVars.lvlib\\stachModeHatchPanelStateMachineControl"(T12."Stach Wait for Gather Extend" ("stachModeHatchPanelStateMachineControl")) -> ()  [unwired: 1 in, 1 out]
              }
            }
            n158 = case shown="True" w259 {
              frame False {
              }
              frame True {
                n159 = shared-variable ".\\hatchPanelSharedVars.lvlib\\stachModeHatchPanelStateMachineControl"(stachModeHatchPanelStatemachineEnum."Stach Closed to Score" ("Hatch Panel State")) -> ()  [unwired: 1 in, 1 out]
              }
            }
            n160 = case shown="True" w263 {
              frame False {
              }
              frame True {
                (unwired) stachModeHatchPanelStatemachineEnum."Stach Wait for Gather Unlock" ("Hatch Panel State")
                n161 = shared-variable ".\\hatchPanelSharedVars.lvlib\\stachModeHatchPanelStateMachineControl"(T12."Stach Wait for Gather Extend" ("stachModeHatchPanelStateMachineControl")) -> ()  [unwired: 1 in, 1 out]
              }
            }
          }
          frame "Stach Wait for Gather Unlock" {
            n162 = shared-variable ".\\hatchPanelSharedVars.lvlib\\hatchPanelSMUnlockTime"() -> (w273:u32)  [unwired: 1 in, 1 out]
            n163 = shared-variable ".\\hatchPanelSharedVars.lvlib\\hatchPanelSMTick"() -> (w276:u32)  [unwired: 1 in, 1 out]
            n164 = Tick Count (ms)() -> (millisecond timer value=w275:u32)
            n165 = Subtract(x=w275, y=w276) -> (x-y=w274:u32)
            n166 = Greater Or Equal?(x=w274, y=w273) -> (x >= y?=w272:bool)
            n167 = case shown="True" w272 {
              frame False {
              }
              frame True {
                n168 = shared-variable ".\\hatchPanelSharedVars.lvlib\\stachModeHatchPanelStateMachineControl"(stachModeHatchPanelStatemachineEnum."Stach Wait for Gather Extend" ("Hatch Panel State")) -> ()  [unwired: 1 in, 1 out]
              }
            }
          }
          frame "Stach Wait for Gather Extend" {
            n169 = shared-variable ".\\hatchPanelSharedVars.lvlib\\hatchPanelSMGatherExtendTime"() -> (w287:u32)  [unwired: 1 in, 1 out]
            n170 = shared-variable ".\\hatchPanelSharedVars.lvlib\\hatchPanelSMTick"() -> (w284:u32)  [unwired: 1 in, 1 out]
            n171 = Tick Count (ms)() -> (millisecond timer value=w285:u32)
            n172 = Subtract(x=w285, y=w284) -> (x-y=w286:u32)
            n173 = Greater Or Equal?(x=w286, y=w287) -> (x >= y?=w283:bool)
            n174 = case shown="True" w283 {
              frame False {
              }
              frame True {
                n175 = shared-variable ".\\hatchPanelSharedVars.lvlib\\stachModeHatchPanelStateMachineControl"(stachModeHatchPanelStatemachineEnum."Stach Gather Extended" ("Hatch Panel State")) -> ()  [unwired: 1 in, 1 out]
              }
            }
          }
          frame "Stach Gather Extended" {
            n176 = call <userlib>:"Stable.vi"("Eval Period (sec)"=0.1, "Signal Input"=w294) -> ("Stable"=w293:bool)  [unwired: 9 in]
            n177 = case shown="True" w298 {
              frame False {
              }
              frame True {
                n178 = shared-variable ".\\hatchPanelSharedVars.lvlib\\stachModeHatchPanelStateMachineControl"(stachModeHatchPanelStatemachineEnum."Stach Wait for Grab Panel" ("Hatch Panel State")) -> ()  [unwired: 1 in, 1 out]
              }
            }
            n179 = case shown="True" w293 {
              frame False {
              }
              frame True {
                n180 = shared-variable ".\\hatchPanelSharedVars.lvlib\\stachModeHatchPanelStateMachineControl"(stachModeHatchPanelStatemachineEnum."Stach Wait for Grab Panel" ("Hatch Panel State")) -> ()  [unwired: 1 in, 1 out]
              }
            }
            n181 = case shown="True" w297 {
              frame False {
              }
              frame True {
                n182 = shared-variable ".\\hatchPanelSharedVars.lvlib\\stachModeHatchPanelStateMachineControl"(stachModeHatchPanelStatemachineEnum."Stach Wait for Score Retract" ("Hatch Panel State")) -> ()  [unwired: 1 in, 1 out]
              }
            }
          }
          frame "Stach Wait for Grab Panel" {
            n183 = disable-structure shown="Disabled" {
              frame Disabled {
                w318 = 0 ("New Position")
                n184 = call <vilib>:"CTRE_Phoenix_MotorControl_RefNumRegistryGet.vi"("refnum name"="leftDrive") -> ("PhoenixMotorControlDevRef"=w317:T20)  [unwired: 9 in, 1 out]
                n185 = call <vilib>:"CTRE_Phoenix_MotorControl_RefNumRegistryGet.vi"("refnum name"="rightDrive") -> ("PhoenixMotorControlDevRef"=w316:T20)  [unwired: 9 in, 1 out]
                n186 = call <vilib>:"CTRE_Phoenix_MotorControl_SetQuadraturePosition_Enhanced.vi"("New Position"=w318, "PhoenixMotorControlDevRef"=w317) -> ()  [unwired: 8 in, 2 out]
                n187 = call <vilib>:"CTRE_Phoenix_MotorControl_SetQuadraturePosition_Enhanced.vi"("New Position"=w318, "PhoenixMotorControlDevRef"=w316) -> ()  [unwired: 8 in, 2 out]
              }
              frame Enabled {
              }
            }
            n188 = shared-variable ".\\hatchPanelSharedVars.lvlib\\hatchPanelSMGrabTime"() -> (w309:u32)  [unwired: 1 in, 1 out]
            n189 = shared-variable ".\\hatchPanelSharedVars.lvlib\\hatchPanelSMTick"() -> (w312:u32)  [unwired: 1 in, 1 out]
            n190 = shared-variable ".\\hatchPanelSharedVars.lvlib\\StoredEncoderValue"(w305) -> ()  [unwired: 1 in, 1 out]
            n191 = Tick Count (ms)() -> (millisecond timer value=w311:u32)
            n192 = Subtract(x=w311, y=w312) -> (x-y=w310:u32)
            n193 = Greater Or Equal?(x=w310, y=w309) -> (x >= y?=w308:bool)
            n194 = case shown="True" w308 {
              frame False {
              }
              frame True {
                n195 = shared-variable ".\\hatchPanelSharedVars.lvlib\\stachModeHatchPanelStateMachineControl"(stachModeHatchPanelStatemachineEnum."Stach Grab Panel" ("Hatch Panel State")) -> ()  [unwired: 1 in, 1 out]
              }
            }
          }
          frame "Stach Grab Panel" {
            n196 = shared-variable ".\\hatchPanelSharedVars.lvlib\\StoredEncoderValue"() -> (w324:dbl)  [unwired: 1 in, 1 out]
            n197 = Subtract(x=w323, y=w324) -> (x-y=w325:dbl)
            "Encoder Inches" <- w325
            n198 = Less Or Equal?(x=w325, y="DistanceWantedAwayFromLoadingStation") -> ()  [unwired: 1 out]
            n199 = case shown="True" w330 {
              frame False {
              }
              frame True {
                n200 = shared-variable ".\\hatchPanelSharedVars.lvlib\\stachModeHatchPanelStateMachineControl"(stachModeHatchPanelStatemachineEnum."Stach Wait for Gather Retract" ("Hatch Panel State")) -> ()  [unwired: 1 in, 1 out]
              }
            }
            n201 = case shown="True" w329 {
              frame False {
              }
              frame True {
                n202 = shared-variable ".\\hatchPanelSharedVars.lvlib\\stachModeHatchPanelStateMachineControl"(stachModeHatchPanelStatemachineEnum."Stach Wait for Gather Extend" ("Hatch Panel State")) -> ()  [unwired: 1 in, 1 out]
              }
            }
            n203 = case shown="True" TRUE {
              frame False {
              }
              frame True {
                n204 = shared-variable ".\\hatchPanelSharedVars.lvlib\\stachModeHatchPanelStateMachineControl"(stachModeHatchPanelStatemachineEnum."Stach Wait for Gather Retract" ("Hatch Panel State")) -> ()  [unwired: 1 in, 1 out]
              }
            }
          }
          frame "Stach Wait for Gather Retract" {
            n205 = shared-variable ".\\hatchPanelSharedVars.lvlib\\hatchPanelSMGatherRetractTime"() -> (w340:u32)  [unwired: 1 in, 1 out]
            n206 = shared-variable ".\\hatchPanelSharedVars.lvlib\\hatchPanelSMTick"() -> (w343:u32)  [unwired: 1 in, 1 out]
            n207 = Tick Count (ms)() -> (millisecond timer value=w342:u32)
            n208 = Subtract(x=w342, y=w343) -> (x-y=w341:u32)
            n209 = Greater Or Equal?(x=w341, y=w340) -> (x >= y?=w339:bool)
            n210 = case shown="True" w339 {
              frame False {
              }
              frame True {
                n211 = shared-variable ".\\hatchPanelSharedVars.lvlib\\stachModeHatchPanelStateMachineControl"(stachModeHatchPanelStatemachineEnum."Stach Closed to Score" ("Hatch Panel State")) -> ()  [unwired: 1 in, 1 out]
              }
            }
          }
          frame "Stach Closed to Score" {
            n212 = Not(x=w353) -> (.not. x?=w351:bool)
            n213 = call <userlib>:"Stable.vi"("Eval Period (sec)"=0.5, "Signal Input"=w351) -> ("Stable"=w350:bool)  [unwired: 9 in]
            n214 = case shown="True" w350 {
              frame False {
              }
              frame True {
                n215 = shared-variable ".\\hatchPanelSharedVars.lvlib\\stachModeHatchPanelStateMachineControl"(stachModeHatchPanelStatemachineEnum."Stach Open to Gather" ("Hatch Panel State")) -> ()  [unwired: 1 in, 1 out]
              }
            }
            n216 = case shown="True" w355 {
              tunnel: [FALSE ("MotionButtonPressedBefore?") TRUE ("MotionButtonPressedBefore?")] -> w354
              frame False {
              }
              frame True {
                (unwired) stachModeHatchPanelStatemachineEnum."Stach Wait for Score Unlock" ("Hatch Panel State")
                n217 = shared-variable ".\\hatchPanelSharedVars.lvlib\\stachModeHatchPanelStateMachineControl"(stachModeHatchPanelStatemachineEnum."Stach Wait for Score Extend" ("Hatch Panel State")) -> ()  [unwired: 1 in, 1 out]
              }
            }
            n218 = case shown="True" w356 {
              frame False {
              }
              frame True {
                n219 = shared-variable ".\\hatchPanelSharedVars.lvlib\\stachModeHatchPanelStateMachineControl"(stachModeHatchPanelStatemachineEnum."Stach Wait for Sonar Signal" ("Hatch Panel State")) -> ()  [unwired: 1 in, 1 out]
              }
            }
            n220 = shared-variable ".\\hatchPanelSharedVars.lvlib\\MotionButtonPressedBefore?"(w354) -> ()  [unwired: 1 in, 1 out]
          }
          frame "Stach Wait for Sonar Signal" {
            n221 = Not(x=w370) -> (.not. x?=w369:bool)
            n222 = Less Or Equal?(x=w365, y="DistanceWantedFromTarget(Inch)") -> (x <= y?=w372:bool)
            n223 = case shown="True" w373 {
              tunnel: [FALSE TRUE] -> w368
              frame False {
              }
              frame True {
                (unwired) stachModeHatchPanelStatemachineEnum."Stach Wait for Score Unlock" ("Hatch Panel State")
                n224 = shared-variable ".\\hatchPanelSharedVars.lvlib\\stachModeHatchPanelStateMachineControl"(stachModeHatchPanelStatemachineEnum."Stach Wait for Score Extend" ("Hatch Panel State")) -> ()  [unwired: 1 in, 1 out]
              }
            }
            n225 = case shown="True" w372 {
              frame False {
              }
              frame True {
                (unwired) stachModeHatchPanelStatemachineEnum."Stach Wait for Score Unlock" ("Hatch Panel State")
                n226 = shared-variable ".\\hatchPanelSharedVars.lvlib\\stachModeHatchPanelStateMachineControl"(stachModeHatchPanelStatemachineEnum."Stach Wait for Score Extend" ("Hatch Panel State")) -> ()  [unwired: 1 in, 1 out]
              }
            }
            n227 = case shown="True" w369 {
              frame False {
              }
              frame True {
                n228 = shared-variable ".\\hatchPanelSharedVars.lvlib\\stachModeHatchPanelStateMachineControl"(stachModeHatchPanelStatemachineEnum."Stach Closed to Score" ("Hatch Panel State")) -> ()  [unwired: 1 in, 1 out]
              }
            }
            n229 = shared-variable ".\\hatchPanelSharedVars.lvlib\\MotionButtonPressedBefore?"(w368) -> ()  [unwired: 1 in, 1 out]
          }
          frame "Stach Wait for Score Unlock" {
            n230 = shared-variable ".\\hatchPanelSharedVars.lvlib\\hatchPanelSMUnlockTime"() -> (w385:u32)  [unwired: 1 in, 1 out]
            n231 = shared-variable ".\\hatchPanelSharedVars.lvlib\\hatchPanelSMTick"() -> (w388:u32)  [unwired: 1 in, 1 out]
            n232 = Tick Count (ms)() -> (millisecond timer value=w387:u32)
            n233 = Subtract(x=w387, y=w388) -> (x-y=w386:u32)
            n234 = Greater Or Equal?(x=w386, y=w385) -> (x >= y?=w384:bool)
            n235 = case shown="True" w384 {
              frame False {
              }
              frame True {
                n236 = shared-variable ".\\hatchPanelSharedVars.lvlib\\stachModeHatchPanelStateMachineControl"(stachModeHatchPanelStatemachineEnum."Stach Wait for Score Extend" ("Hatch Panel State")) -> ()  [unwired: 1 in, 1 out]
              }
            }
          }
          frame "Stach Wait for Score Extend" {
            n237 = shared-variable ".\\hatchPanelSharedVars.lvlib\\hatchPanelSMScoreExtendTime"() -> (w396:u32)  [unwired: 1 in, 1 out]
            n238 = shared-variable ".\\hatchPanelSharedVars.lvlib\\hatchPanelSMTick"() -> (w399:u32)  [unwired: 1 in, 1 out]
            n239 = Tick Count (ms)() -> (millisecond timer value=w398:u32)
            n240 = Subtract(x=w398, y=w399) -> (x-y=w397:u32)
            n241 = Greater Or Equal?(x=w397, y=w396) -> (x >= y?=w395:bool)
            n242 = case shown="True" w395 {
              frame False {
              }
              frame True {
                n243 = shared-variable ".\\hatchPanelSharedVars.lvlib\\MotionButtonPressedBefore?"() -> (w403:bool)  [unwired: 1 in, 1 out]
                n244 = case shown="False" w403 {
                  frame False {
                    n245 = shared-variable ".\\hatchPanelSharedVars.lvlib\\stachModeHatchPanelStateMachineControl"(stachModeHatchPanelStatemachineEnum."Stach Wait for Release Panel" ("Hatch Panel State")) -> ()  [unwired: 1 in, 1 out]
                  }
                  frame True {
                    n246 = shared-variable ".\\hatchPanelSharedVars.lvlib\\stachModeHatchPanelStateMachineControl"(stachModeHatchPanelStatemachineEnum."Stach Ready to Score " ("Hatch Panel State")) -> ()  [unwired: 1 in, 1 out]
                  }
                }
              }
            }
          }
          frame "Stach Ready to Score " {
            n247 = case shown="True" w409 {
              frame False {
              }
              frame True {
                n248 = shared-variable ".\\hatchPanelSharedVars.lvlib\\stachModeHatchPanelStateMachineControl"(stachModeHatchPanelStatemachineEnum."Stach Wait for Gather Retract" ("Hatch Panel State")) -> ()  [unwired: 1 in, 1 out]
              }
            }
            n249 = case shown="True" w406 {
              frame False {
              }
              frame True {
                n250 = shared-variable ".\\hatchPanelSharedVars.lvlib\\stachModeHatchPanelStateMachineControl"(stachModeHatchPanelStatemachineEnum."Stach Wait for Release Panel" ("Hatch Panel State")) -> ()  [unwired: 1 in, 1 out]
              }
            }
          }
          frame "Stach Wait for Release Panel" {
            n251 = shared-variable ".\\hatchPanelSharedVars.lvlib\\hatchPanelSMReleaseTime"() -> (w418:u32)  [unwired: 1 in, 1 out]
            n252 = shared-variable ".\\hatchPanelSharedVars.lvlib\\hatchPanelSMTick"() -> (w421:u32)  [unwired: 1 in, 1 out]
            n253 = Tick Count (ms)() -> (millisecond timer value=w420:u32)
            n254 = Subtract(x=w420, y=w421) -> (x-y=w419:u32)
            n255 = Greater Or Equal?(x=w419, y=w418) -> (x >= y?=w417:bool)
            n256 = case shown="True" w417 {
              frame False {
              }
              frame True {
                n257 = shared-variable ".\\hatchPanelSharedVars.lvlib\\stachModeHatchPanelStateMachineControl"(stachModeHatchPanelStatemachineEnum."Stach Release Panel" ("Hatch Panel State")) -> ()  [unwired: 1 in, 1 out]
              }
            }
          }
          frame "Stach Release Panel" {
            n258 = shared-variable ".\\hatchPanelSharedVars.lvlib\\stachModeHatchPanelStateMachineControl"(stachModeHatchPanelStatemachineEnum."Stach Wait for Score Retract" ("Hatch Panel State")) -> ()  [unwired: 1 in, 1 out]
          }
          frame "Stach Wait for Score Retract" {
            n259 = shared-variable ".\\hatchPanelSharedVars.lvlib\\hatchPanelSMScoreRetractTime"() -> (w435:u32)  [unwired: 1 in, 1 out]
            n260 = shared-variable ".\\hatchPanelSharedVars.lvlib\\hatchPanelSMTick"() -> (w438:u32)  [unwired: 1 in, 1 out]
            n261 = Tick Count (ms)() -> (millisecond timer value=w437:u32)
            n262 = Subtract(x=w437, y=w438) -> (x-y=w436:u32)
            n263 = Greater Or Equal?(x=w436, y=w435) -> (x >= y?=w434:bool)
            n264 = case shown="True" w434 {
              frame False {
              }
              frame True {
                n265 = shared-variable ".\\hatchPanelSharedVars.lvlib\\stachModeHatchPanelStateMachineControl"(stachModeHatchPanelStatemachineEnum."Stach Open to Gather" ("Hatch Panel State")) -> ()  [unwired: 1 in, 1 out]
              }
            }
          }
        }
        n266 = feedback #4(stachModeHatchPanelStatemachineEnum."Stach Closed to Score" ("Hatch Panel State")) -> (w247:T12)
        n267 = feedback-in #4(w240) -> ()
        n268 = Not Equal?(x=w240, y=w247) -> (x != y?=w248:bool)
        n269 = case shown="True" w248 {
          frame False {
          }
          frame True {
            n270 = Tick Count (ms)() -> (millisecond timer value=w256:u32)
            n271 = shared-variable ".\\hatchPanelSharedVars.lvlib\\hatchPanelSMTick"(w256) -> ()  [unwired: 1 in, 1 out]
          }
        }
        n272 = disable-structure shown="Disabled" {
          disable-tunnel: w240 -> [w255 _]
          frame Disabled {
            n273 = shared-variable ".\\TDMS.lvlib\\TDMS DevRef"() -> (w253:T15)  [unwired: 1 in, 1 out]
            n274 = call <userlib>:"Logger_Log_Data.vi"("Data"=w255, "Channel"="Hatch_Panel_Stach_State", "Group"="Robot_Data", "TDMS DevRef"=w253) -> ()  [unwired: 7 in, 1 out]
          }
          frame Enabled {
          }
        }
      }
      frame "Climb Mode" {
        n275 = Equal?(x=w446, y=HatchPanelMotionEnum."Extend") -> (x = y?=w444:bool)
        n276 = Select(t=hatchPanelClimbSMEnum."Ready for Climb", s=w444, f=hatchPanelClimbSMEnum."Start") -> (s? t:f=w449:T13)
        n277 = feedback #5() -> (w460:T13)  [unwired: 1 in]
        n278 = feedback #6() -> (w457:u32)  [unwired: 1 in]
        n279 = feedback #7(hatchPanelClimbSMEnum."Start") -> (w459:T13)
        n280 = feedback-in #5(w459) -> ()
        n281 = Select(t=w449, s=w455, f=w459) -> (s? t:f=w450:T13)
        n282 = disable-structure shown="Disabled" {
          disable-tunnel: w450 -> [w466 _]
          frame Disabled {
            n283 = shared-variable ".\\TDMS.lvlib\\TDMS DevRef"() -> (w464:T15)  [unwired: 1 in, 1 out]
            n284 = call <userlib>:"Logger_Log_Data.vi"("Data"=w466, "Channel"="Hatch_Panel_Climb_Mode_State", "Group"="Robot_Data", "TDMS DevRef"=w464) -> ()  [unwired: 7 in, 1 out]
          }
          frame Enabled {
          }
        }
        n285 = Not Equal?(x=w459, y=w460) -> (x != y?=w458:bool)
        n286 = case shown="True" w458 {
          tunnel: [w467 w468] -> w456
          tunnel: w457 -> [w467 _]
          frame False {
          }
          frame True {
            n287 = Tick Count (ms)() -> (millisecond timer value=w468:u32)
          }
        }
        n288 = feedback-in #6(w456) -> ()
        n289 = case shown="\"Finished Climb\"" w450 {
          selector: w450 -> [_ w475 w488 w503 _]
          tunnel: [hatchPanelClimbSMEnum."Unlock" w476 w489 w502 hatchPanelClimbSMEnum."Finished Climb" ("t")] -> w462
          tunnel: [hatchPanelLockEnum."Unlocked" hatchPanelLockEnum."Unlocked" hatchPanelLockEnum."Unlocked" hatchPanelLockEnum."Unlocked" hatchPanelLockEnum."Unlocked"] -> w452
          tunnel: [HatchGrabPistonEnum."Close" HatchGrabPistonEnum."Close" HatchGrabPistonEnum."Close" HatchGrabPistonEnum."Close" HatchGrabPistonEnum."Close"] -> w453
          tunnel: [HatchPanelMotionEnum."Retract" HatchPanelMotionEnum."Retract" HatchPanelMotionEnum."Extend" HatchPanelMotionEnum."Extend" HatchPanelMotionEnum."Retract"] -> w454
          tunnel: w456 -> [_ w479 w492 _ _]
          tunnel: [FALSE FALSE FALSE TRUE FALSE] -> w451
          frame "Start", Default {
          }
          frame "Unlock" {
            n290 = Add(x=w479, y="Wait for Unlock Time (ms)") -> (x+y=w480:u32)
            n291 = Tick Count (ms)() -> (millisecond timer value=w481:u32)
            n292 = Greater Or Equal?(x=w481, y=w480) -> (x >= y?=w477:bool)
            n293 = case shown="False" w477 {
              tunnel: [w485 hatchPanelClimbSMEnum."Extend"] -> w476
              tunnel: w475 -> [w485 _]
              frame False {
              }
              frame True {
              }
            }
          }
          frame "Extend" {
            n294 = Add(x=w492, y="Wait for Extend Time (ms)") -> (x+y=w493:u32)
            n295 = Tick Count (ms)() -> (millisecond timer value=w494:u32)
            n296 = Greater Or Equal?(x=w494, y=w493) -> (x >= y?=w490:bool)
            n297 = case shown="True" w490 {
              tunnel: [w498 hatchPanelClimbSMEnum."Ready for Climb"] -> w489
              tunnel: w488 -> [w498 _]
              frame False {
              }
              frame True {
              }
            }
          }
          frame "Ready for Climb" {
            n298 = shared-variable ".\\climbSharedVars.lvlib\\climbFinished"() -> (w501:bool)  [unwired: 1 in, 1 out]
            n299 = Select(t=hatchPanelClimbSMEnum."Finished Climb", s=w501, f=w503) -> (s? t:f=w502:T13)
          }
          frame "Finished Climb" {
          }
        }
        n300 = feedback-in #7(w462) -> ()
      }
      frame "Retracted Closed" {
      }
      frame "Retracted Open" {
      }
      frame "Extended Closed" {
      }
      frame "Extended Open" {
      }
    }
    n301 = feedback-in #2(w23) -> ()
    n302 = shared-variable ".\\hatchPanelSharedVars.lvlib\\hatchPanelSMGrabTime"("hatchPanelSMGrabTime") -> ()  [unwired: 1 in, 1 out]
    n303 = shared-variable ".\\ControlRoom.lvlib\\HatchPannelPeriod"() -> (w25:i64)  [unwired: 1 in, 1 out]
    n304 = Unbundle By Name(w17) -> ("Hatch Panel State"=w16:T8)
    n305 = disable-structure shown="Disabled" {
      disable-tunnel: w25 -> [w56 _]
      frame Disabled {
        n306 = shared-variable ".\\TDMS.lvlib\\TDMS DevRef"() -> (w54:T15)  [unwired: 1 in, 1 out]
        n307 = call <userlib>:"Logger_Log_Data.vi"("Data"=w56, "Channel"="Hatch_Panel_Loop_Period", "Group"="Robot_Data", "TDMS DevRef"=w54) -> ()  [unwired: 7 in, 1 out]
      }
      frame Enabled {
      }
    }
    n308 = shared-variable ".\\hatchPanelSharedVars.lvlib\\hatchPanelReadyForClimb"(w28) -> ()  [unwired: 1 in, 1 out]
    n309 = shared-variable ".\\hatchPanelSharedVars.lvlib\\hatchPanelScored"(w9) -> ()  [unwired: 1 in, 1 out]
    n310 = disable-structure shown="Disabled" {
      disable-tunnel: w16 -> [w52 _]
      frame Disabled {
        n311 = shared-variable ".\\TDMS.lvlib\\TDMS DevRef"() -> (w50:T15)  [unwired: 1 in, 1 out]
        n312 = call <userlib>:"Logger_Log_Data.vi"("Data"=w52, "Channel"="Hatch_Panel_State", "Group"="Robot_Data", "TDMS DevRef"=w50) -> ()  [unwired: 7 in, 1 out]
      }
      frame Enabled {
      }
    }
    n313 = call "hatchPanelMotion.vi"(10:w23, "Extend SolenoidDevRef"=w12) -> ()  [unwired: 10 in]
    n314 = call "hatchGrabPiston.vi"("Enum"=w13, "Grab SolenoidDevRef"=w11) -> ()  [unwired: 10 in]
    n315 = call "hatchPanelLock.vi"(10:w36, "Lock SolenoidDevRef"=w10) -> ()  [unwired: 10 in]
    n316 = Equal?(x=w13, y=HatchGrabPistonEnum."Close") -> (x = y?=w15:bool)
    n317 = shared-variable ".\\hatchPanelSharedVars.lvlib\\Hatch_Claws_Close?"(w15) -> ()  [unwired: 1 in, 1 out]
    n318 = node-c288(w25) -> ()  [unwired: 1 out]
  }
  n319 = node-c288(w7) -> ()  [unwired: 1 out]
